vi "Auto Analysis.vi"(8 "error in (no error)":errorcluster, 11 "NRT8000 in":refnum<class "NRT8000.lvclass">) -> (0 "error out":errorcluster, 2 "Analysis Data":T1, 3 "NRT8000 out":refnum<class "NRT8000.lvclass">)   [LabVIEW 2018, in "NRT8000.lvlib" / "NRT8000.lvclass"]
uses:
  NRT8000.lvclass
  PPLs/Optical Spectrum Analyzer/Parent/OSA.lvlibp/Custom Controls/Analysis Data.ctl
  PPLs/Optical Spectrum Analyzer/Parent/OSA.lvlibp/Optical Spectrum Analyzer.lvclass
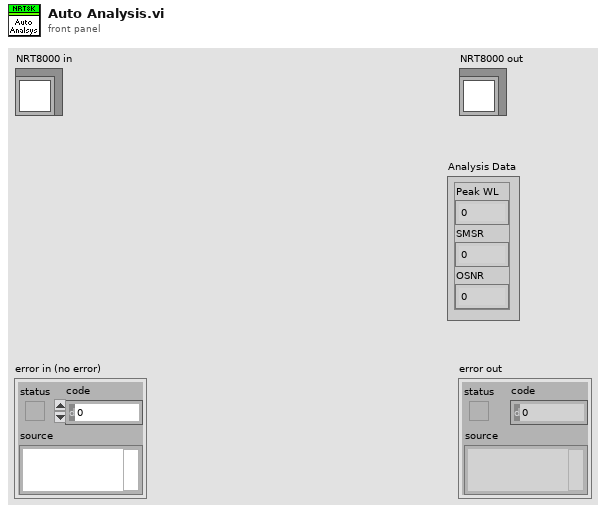
[diagram p1: front panel]
types:
  T1 = typedef "OSA.lvlibp/Optical Spectrum Analyzer.lvclass/Analysis Data.ctl" = cluster{"Peak WL":dbl, "SMSR":dbl, "OSNR":dbl}
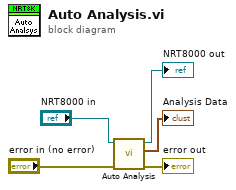
[diagram p0: block diagram]
diagram:
  n1 = call-parent "Auto Analysis.vi"("error in (no error)"="error in (no error)", "Optical Spectrum Analyzer in"="NRT8000 in") -> ("error out"=→"error out":errorcluster, "Analysis Data"=→"Analysis Data":T1, "Optical Spectrum Analyzer out"=→"NRT8000 out":refnum<class "NRT8000.lvclass">)  [unwired: 7 in]
